vi "LakeShore Ramp Text Out.vi"(1 "LSRamp":T1={"VISA Resource Name"="", "extra wait"=0, "start (K/W)"=1e-09, "end (K/W)"=0.001, "Sweep Time (H:M:S)"=3600.0, "Mapping"=FALSE, "Parameter"=FALSE, "Loop"=FALSE} {"Sweep Time (H:M:S)" format="%<%H:%M:%S>t"; "extra wait" min=0; "start (K/W)" format="%#.7e"; "end (K/W)" format="%#.7e"}) -> (0 "Command text":string[][](array[string]))   [LabVIEW 2019]
uses:
  LSRamp.ctl
panel:
  out "Sweep Time (H:M:S)":dbl
  out "String Cluster":T2
  # "LakeShore Ramp"
  # "Log"
  # "Start Temp(K)/Power(W)"
  # "Sweep Time (HH:MM:SS)"
  # "End Temp(K)/Power(W)"
  # "Linear"
  # "seconds"
  # "AND wait extra"
  # "Power"
  # "Temp"
  # "VISA Name"
  # "Loop 2"
  # "Loop 1"
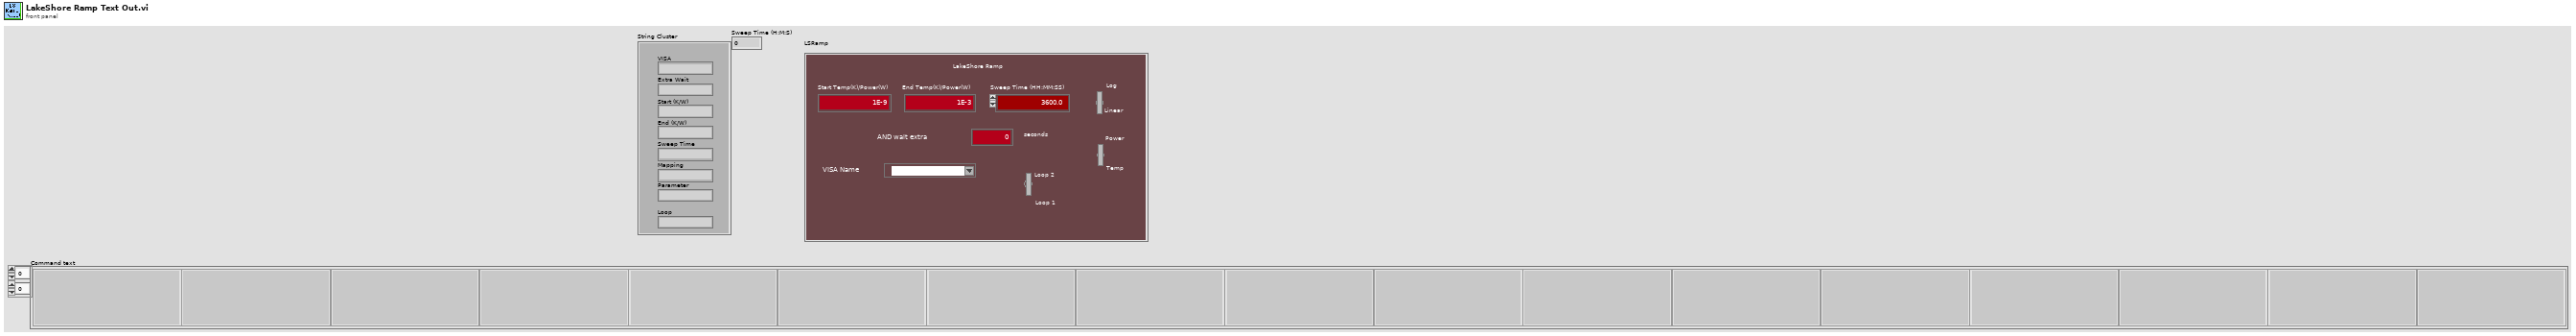
[diagram p1: front panel]
types:
  T1 = typedef "LSRamp.ctl" = cluster{"VISA Resource Name":refnum<visa-resource-name>, "extra wait":i32, "start (K/W)":dbl, "end (K/W)":dbl, "Sweep Time (H:M:S)":dbl, "Mapping":bool, "Parameter":bool, "Loop":bool}
  T2 = cluster{"VISA":string, "Extra Wait":string, "Start (K/W)":string, "End (K/W)":string, "Sweep Time":string, "Mapping":string, "Parameter":string, "Loop":string}
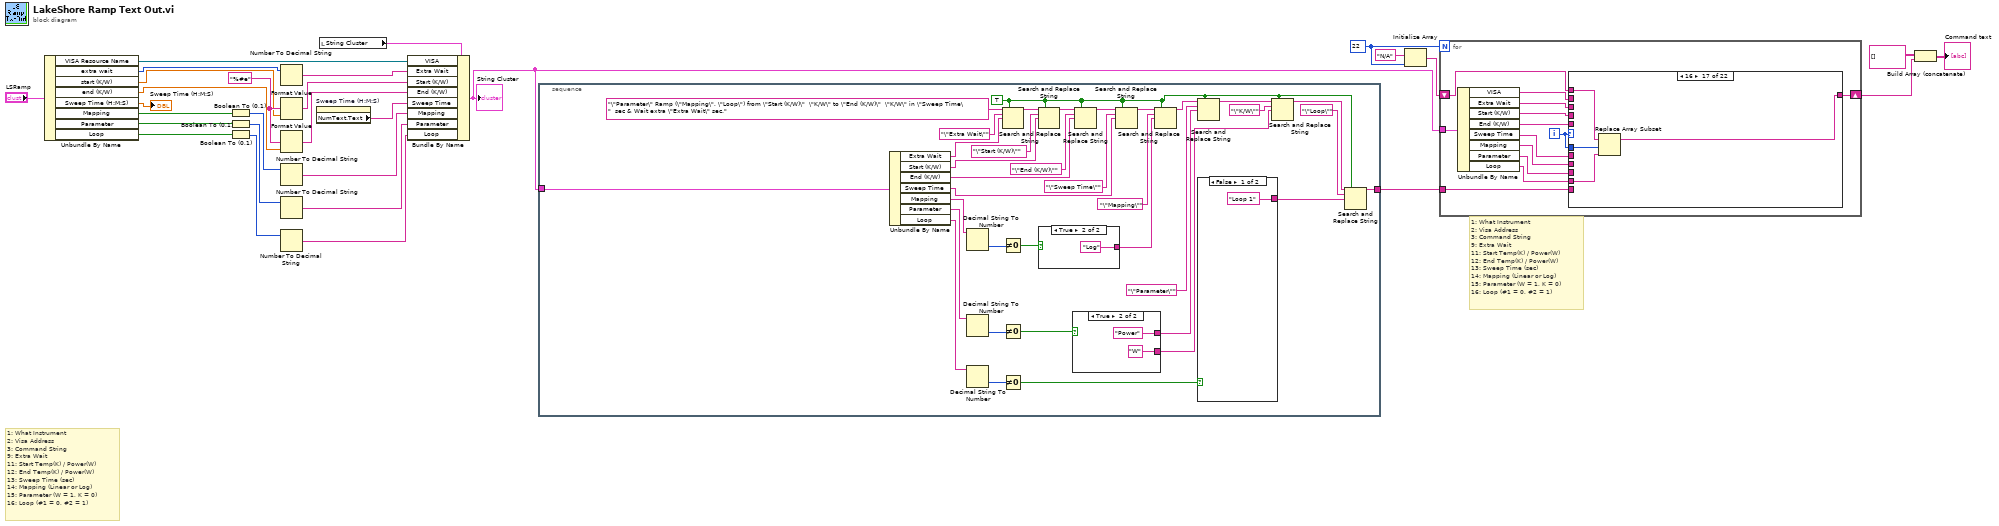
[diagram p0: block diagram]
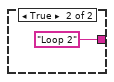
[diagram p2: hidden frame]
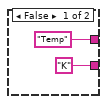
[diagram p3: hidden frame]
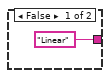
[diagram p4: hidden frame]
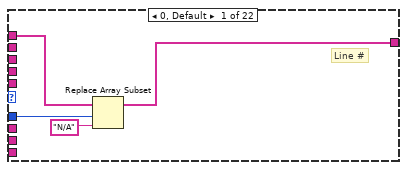
[diagram p5: hidden frame]
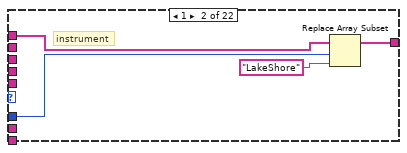
[diagram p6: hidden frame]
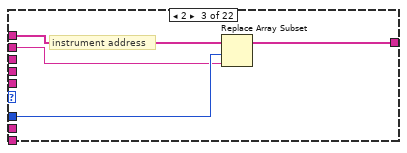
[diagram p7: hidden frame]
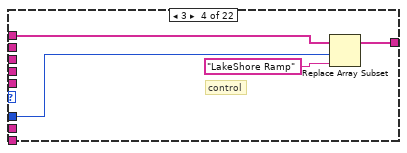
[diagram p8: hidden frame]
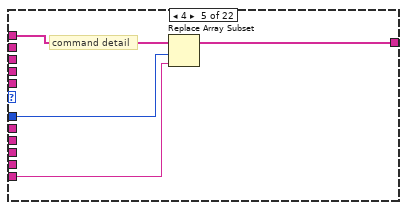
[diagram p9: hidden frame]
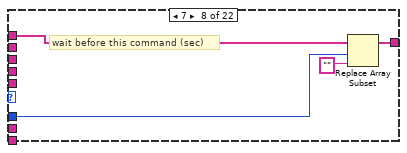
[diagram p12: hidden frame]
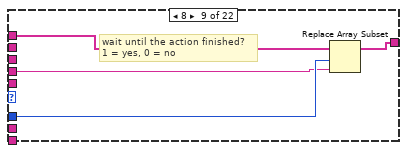
[diagram p13: hidden frame]
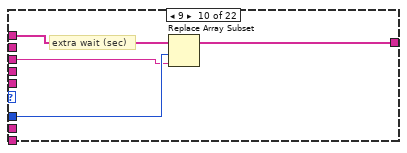
[diagram p14: hidden frame]
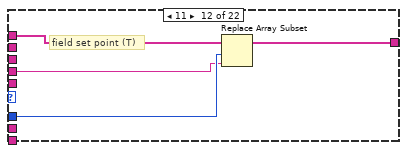
[diagram p16: hidden frame]
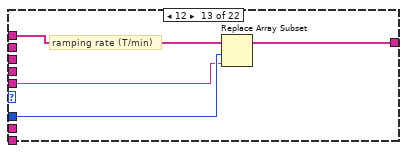
[diagram p17: hidden frame]
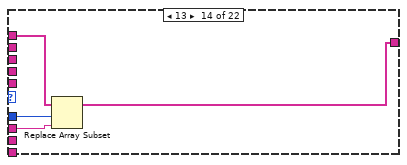
[diagram p18: hidden frame]
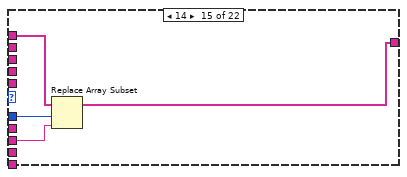
[diagram p19: hidden frame]
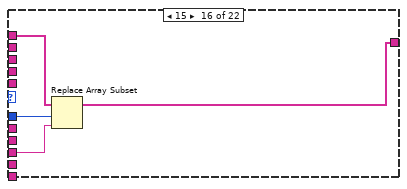
[diagram p20: hidden frame]
diagram:
  w18 = "%#e" ("format string")
  w26 = 22
  # "1: What Instrument\n2: Visa Address\n3: Command String\n9: Extra Wait\n11: Start Temp(K) / Power(W)\n12: End Temp(K) / Power(W)\n13: Sweep Time (sec)\n14: Mapping (Linear or Log)\n15: Parameter (W = 1, K = 0)\n16: Loop (#1 = 0, #2 = 1)"
  # "1: What Instrument\n2: Visa Address\n3: Command String\n9: Extra Wait\n11: Start Temp(K) / Power(W)\n12: End Temp(K) / Power(W)\n13: Sweep Time (sec)\n14: Mapping (Linear or Log)\n15: Parameter (W = 1, K = 0)\n16: Loop (#1 = 0, #2 = 1)"
  n1 = Unbundle By Name("LSRamp") -> ("VISA Resource Name"=w11:refnum<visa-resource-name>, "extra wait"=w13:i32, "start (K/W)"=w16:dbl, "end (K/W)"=w17:dbl, "Sweep Time (H:M:S)"=→"Sweep Time (H:M:S)":dbl, "Mapping"=w9:bool, "Parameter"=w4:bool, "Loop"=w3:bool)
  n2 = Boolean To (0,1)(Boolean=w9) -> (0, 1=w10:i16)
  n3 = Boolean To (0,1)(Boolean=w4) -> (0, 1=w2:i16)
  n4 = Boolean To (0,1)(Boolean=w3) -> (0, 1=w1:i16)
  n5 = Number To Decimal String(number=w13) -> (decimal integer string=w12:string)  [unwired: 1 in]
  n6 = Format Value(format string=w18, value (0)=w16) -> (output string=w15:string)  [unwired: 1 in]
  n7 = Format Value(format string=w18, value (0)=w17) -> (output string=w14:string)  [unwired: 1 in]
  n8 = Number To Decimal String(number=w10) -> (decimal integer string=w8:string)  [unwired: 1 in]
  n9 = Number To Decimal String(number=w2) -> (decimal integer string=w5:string)  [unwired: 1 in]
  n10 = Number To Decimal String(number=w1) -> (decimal integer string=w6:string)  [unwired: 1 in]
  n11 = property on="Sweep Time (H:M:S)" class="DigNum (strict)"() -> ("NumText.Text"=w19:string)  [unwired: 2 in, 2 out]
  n12 = local read "String Cluster"() -> (w23:T2)
  n13 = Bundle By Name(cluster=w23, "VISA"=w11, "Extra Wait"=w12, "Start (K/W)"=w15, "End (K/W)"=w14, "Sweep Time"=w19, "Mapping"=w8, "Parameter"=w5, "Loop"=w6) -> (w21:T2)
  "String Cluster" <- w21
  n14 = stacked-sequence {
    tunnel: [w31] -> w22
    tunnel: w21 -> [w57]
    frame #0 {
      w30 = TRUE
      n15 = Unbundle By Name(w57) -> ("Extra Wait"=w56:string, "Start (K/W)"=w55:string, "End (K/W)"=w54:string, "Sweep Time"=w53:string, "Mapping"=w41:string, "Parameter"=w40:string, "Loop"=w39:string)
      n16 = Decimal String To Number(string=w41) -> (number=w47:i32)  [unwired: 2 in, 1 out]
      n17 = Decimal String To Number(string=w40) -> (number=w46:i32)  [unwired: 2 in, 1 out]
      n18 = Decimal String To Number(string=w39) -> (number=w45:i32)  [unwired: 2 in, 1 out]
      n19 = Search and Replace String(replace all?=w30, input string="\"Parameter\" Ramp (\"Mapping\", \"Loop\") from \"Start (K/W)\"  \"K/W\" to \"End (K/W)\"  \"K/W\" in \"Sweep Time\"  sec & Wait extra \"Extra Wait\" sec.", search string="\"Extra Wait\"", replace string=w56) -> (result string=w63:string)  [unwired: 4 in, 3 out]
      n20 = Not Equal To 0?(x=w47) -> (x != 0?=w44:bool)
      n21 = Not Equal To 0?(x=w46) -> (x != 0?=w43:bool)
      n22 = Not Equal To 0?(x=w45) -> (x != 0?=w42:bool)
      n23 = Search and Replace String(replace all?=w30, input string=w63, search string="\"Start (K/W)\"", replace string=w55) -> (result string=w64:string)  [unwired: 4 in, 3 out]
      n24 = case shown="True" w44 {
        tunnel: ["Linear" "Log"] -> w52
        frame False {
        }
        frame True {
        }
      }
      n25 = case shown="True" w43 {
        tunnel: ["Temp" "Power"] -> w38
        tunnel: ["K" "W"] -> w35
        frame False {
        }
        frame True {
        }
      }
      n26 = Search and Replace String(replace all?=w30, input string=w64, search string="\"End (K/W)\"", replace string=w54) -> (result string=w65:string)  [unwired: 4 in, 3 out]
      n27 = Search and Replace String(replace all?=w30, input string=w65, search string="\"Sweep Time\"", replace string=w53) -> (result string=w51:string)  [unwired: 4 in, 3 out]
      n28 = Search and Replace String(replace all?=w30, input string=w51, search string="\"Mapping\"", replace string=w52) -> (result string=w48:string)  [unwired: 4 in, 3 out]
      n29 = Search and Replace String(replace all?=w30, input string=w48, search string="\"Parameter\"", replace string=w38) -> (result string=w37:string)  [unwired: 4 in, 3 out]
      n30 = case shown="False" w42 {
        tunnel: ["Loop 1" "Loop 2"] -> w32
        frame False {
        }
        frame True {
        }
      }
      n31 = Search and Replace String(replace all?=w30, input string=w37, search string="\"K/W\"", replace string=w35) -> (result string=w33:string)  [unwired: 4 in, 3 out]
      n32 = Search and Replace String(replace all?=w30, input string=w33, search string="\"Loop\"", replace string=w32) -> (result string=w31:string)  [unwired: 4 in, 3 out]
    }
  }
  n33 = Initialize Array("N/A", w26) -> (w25:string[])
  n34 = for {
    N: w26 -> [_]
    shift-right: [w84] -> w24
    shift-left: w25 -> [w85]
    tunnel: w22 -> [w83]
    tunnel: w21 -> [w82]
    i -> [w86]
    n35 = Unbundle By Name(w82) -> ("VISA"=w79:string, "Extra Wait"=w78:string, "Start (K/W)"=w81:string, "End (K/W)"=w80:string, "Sweep Time"=w77:string, "Mapping"=w76:string, "Parameter"=w75:string, "Loop"=w74:string)
    n36 = case shown="16" w86 {
      tunnel: w86 -> [w89 w93 w98 w100 w105 _ _ w110 w114 w118 _ w123 w127 w133 w135 w139 w143 _ _ _ _ _]
      tunnel: w85 -> [w90 w92 w97 w101 w106 w107 w108 w112 w116 w120 w121 w124 w129 w131 w137 w141 w145 w146 w147 w148 w149 w150]
      tunnel: [w87 w91 w96 w99 w104 w107 w108 w111 w115 w119 w121 w125 w128 w130 w136 w140 w144 w146 w147 w148 w149 w150] -> w84
      tunnel: w83 -> [_ _ _ _ w103 _ _ _ _ _ _ _ _ _ _ _ _ _ _ _ _ _]
      tunnel: w81 -> [_ _ _ _ _ _ _ _ w113 _ _ w122 _ _ _ _ _ _ _ _ _ _]
      tunnel: w80 -> [_ _ _ _ _ _ _ _ _ _ _ _ w126 _ _ _ _ _ _ _ _ _]
      tunnel: w79 -> [_ _ w95 _ _ _ _ _ _ _ _ _ _ _ _ _ _ _ _ _ _ _]
      tunnel: w78 -> [_ _ _ _ _ _ _ _ _ w117 _ _ _ _ _ _ _ _ _ _ _ _]
      tunnel: w77 -> [_ _ _ _ _ _ _ _ _ _ _ _ _ w132 _ _ _ _ _ _ _ _]
      tunnel: w76 -> [_ _ _ _ _ _ _ _ _ _ _ _ _ _ w134 _ _ _ _ _ _ _]
      tunnel: w75 -> [_ _ _ _ _ _ _ _ _ _ _ _ _ _ _ w138 _ _ _ _ _ _]
      tunnel: w74 -> [_ _ _ _ _ _ _ _ _ _ _ _ _ _ _ _ w142 _ _ _ _ _]
      frame 0, Default {
        # "Line #"
        n37 = Replace Array Subset(array=w90, new element="N/A", index=w89) -> (w87:string[])
      }
      frame 1 {
        # "instrument"
        n38 = Replace Array Subset(array=w92, new element="LakeShore", index=w93) -> (w91:string[])
      }
      frame 2 {
        # "instrument address"
        n39 = Replace Array Subset(array=w97, new element=w95, index=w98) -> (w96:string[])
      }
      frame 3 {
        # "control"
        n40 = Replace Array Subset(array=w101, new element="LakeShore Ramp", index=w100) -> (w99:string[])
      }
      frame 4 {
        # "command detail"
        n41 = Replace Array Subset(array=w106, new element=w103, index=w105) -> (w104:string[])
      }
      frame 5 {
        # "in  case 1"
      }
      frame 6 {
        # "in case 2"
      }
      frame 7 {
        # "wait before this command (sec)"
        n42 = Replace Array Subset(array=w112, new element="" ("new element/subarray"), index=w110) -> (w111:string[])
      }
      frame 8 {
        # "wait until the action finished?\n1 = yes, 0 = no"
        n43 = Replace Array Subset(array=w116, new element=w113, index=w114) -> (w115:string[])
      }
      frame 9 {
        # "extra wait (sec)"
        n44 = Replace Array Subset(array=w120, new element=w117, index=w118) -> (w119:string[])
      }
      frame 10 {
      }
      frame 11 {
        # "field set point (T)"
        n45 = Replace Array Subset(array=w124, new element=w122, index=w123) -> (w125:string[])
      }
      frame 12 {
        # "ramping rate (T/min)"
        n46 = Replace Array Subset(array=w129, new element=w126, index=w127) -> (w128:string[])
      }
      frame 13 {
        n47 = Replace Array Subset(array=w131, new element=w132, index=w133) -> (w130:string[])
      }
      frame 14 {
        n48 = Replace Array Subset(array=w137, new element=w134, index=w135) -> (w136:string[])
      }
      frame 15 {
        n49 = Replace Array Subset(array=w141, new element=w138, index=w139) -> (w140:string[])
      }
      frame 16 {
        n50 = Replace Array Subset(array=w145, new element=w142, index=w143) -> (w144:string[])
      }
      frame 17 {
      }
      frame 18 {
      }
      frame 19 {
      }
      frame 20 {
      }
      frame 21 {
      }
    }
  }
  n51 = Build Array (concatenate)(string[][] [], w24) -> (→"Command text":string[][])
